vi "Read All.vi"(8 "error in":errorcluster, 11 "VISA resource name":refnum<visa-resource-name>) -> (0 "error out":errorcluster, 1 "Length":u32, 2 "Message":string, 3 "VISA resource name out":refnum<visa-resource-name>)   [LabVIEW 2017, in "Andeen-Hagerling 2700.lvlib"]
doc: "Read all characters until from the selected VISA resource until no more are available. There is a 100 ms delay before each poll to allow for delays in the bridge. This is allows multiline results to be read completely."
uses:
  Andeen-Hagerling 2700.lvlib
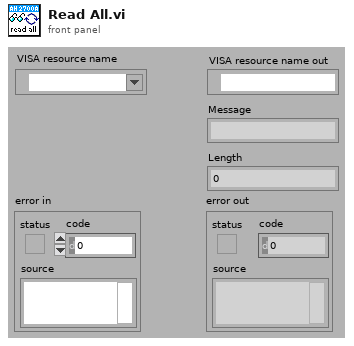
[diagram p1: front panel]
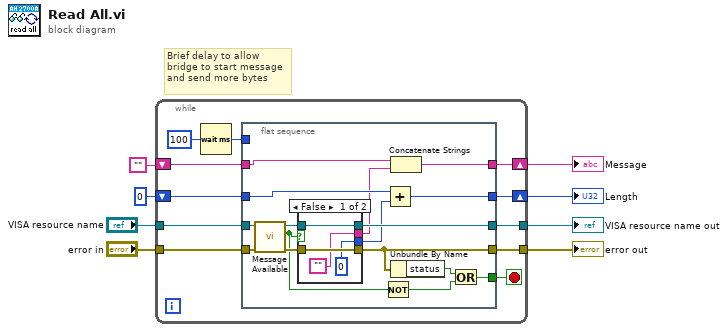
[diagram p0: block diagram]
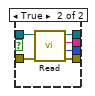
[diagram p2: hidden frame]
diagram:
  # "Brief delay to allow\nbridge to start message\nand send more bytes"
  n1 = while {
    tunnel: "error in" -> [w19]
    tunnel: "VISA resource name" -> [w18]
    tunnel: [w16] -> w4
    tunnel: [w17] -> w3
    shift-right: [w15] -> w2
    shift-left: u32 0 -> [w14]
    shift-right: [w12] -> w1
    shift-left: "" -> [w13]
    stop <- w11 stop-if-true
    n2 = Wait (ms)(milliseconds to wait=u32 100) -> (millisecond timer value=w9:u32)
    n3 = flat-sequence {
      tunnel: w19 -> [w35]
      tunnel: w18 -> [w34]
      tunnel: [w31] -> w17
      tunnel: [w20] -> w16
      tunnel: [w29] -> w15
      tunnel: w14 -> [w28]
      tunnel: w13 -> [w26]
      tunnel: [w25] -> w12
      tunnel: [w21] -> w11
      tunnel: w9 -> [_]
      frame #0 {
        n4 = call "Message Available.vi"("error in"=w35, "VISA resource name"=w34) -> ("error out"=w32:errorcluster, "message available"=w23:bool, "VISA resource name out"=w33:refnum<visa-resource-name>)  [unwired: 7 in]
        n5 = case shown="False" w23 {
          tunnel: w33 -> [w39 w45]
          tunnel: w32 -> [w38 w44]
          tunnel: [u32 0 ("Length") w43] -> w30
          tunnel: ["" w42] -> w27
          tunnel: [w39 w41] -> w31
          tunnel: [w38 w40] -> w20
          frame False {
          }
          frame True {
            n6 = call "Read.vi"("error in"=w44, "VISA resource name"=w45) -> ("error out"=w40:errorcluster, "Length"=w43:u32, "Message"=w42:string, "VISA resource name out"=w41:refnum<visa-resource-name>)  [unwired: 6 in]
          }
        }
        n7 = Not(x=w23) -> (.not. x?=w22:bool)
        n8 = Add(x=w28, y=w30) -> (x+y=w29:u32)
        n9 = Concatenate Strings(w26, w27) -> (w25:string)
        n10 = Unbundle By Name(w20) -> ("status"=w24:bool)
        n11 = Or(x=w24, y=w22) -> (x .or. y?=w21:bool)
      }
    }
  }
  "VISA resource name out" <- w3
  "error out" <- w4
  "Message" <- w1
  "Length" <- w2
